vi "Audio Analysis.vi"() -> ()   [LabVIEW 2023]
doc: "演示在LabVIEW中使用队列消息处理器设计模式的基本概念。最简单的队列消息处理器由2个循环组成。“事件处理”循环通过消息队列，将用户界面事件排序为消息队列。这些消息在“消息处理”循环中出队列。注意，“消息处理”循环可以发送消息到自身。"
uses:
  Ctl/QMH Fundamentals - Message Cluster.ctl
  <vilib>/sound2/lvsound2.llb/Sampling Mode.ctl
  <vilib>/sound2/lvsound2.llb/Sound Data Format.ctl
  <vilib>/Analysis/3filter.llb/Filter Passband Type.ctl
  <vilib>/Analysis/5stat.llb/RMS (DBL).vi
  <vilib>/sound2/lvsound2.llb/Sound File Write Open.vi
  <vilib>/sound2/lvsound2.llb/Sound Input Read (DBL).vi
  <vilib>/sound2/lvsound2.llb/Sound File Write (DBL).vi
  <vilib>/Analysis/3filter.llb/Butterworth Filter (DBL).vi
  <vilib>/Analysis/NI_AALPro.lvlib
  <vilib>/Analysis/NI_AALBase.lvlib
  <vilib>/sound2/lvsound2.llb/Sound Output Write (DBL Single).vi
  <vilib>/sound2/lvsound2.llb/Sound Output Write (DBL).vi
panel:
  out "滤波后频谱图":cluster{"f0":dbl, "df":dbl, "magnitude":dbl[]}(graph) caption="波形图 2"
  out "滤波后信号":waveform(dbl)(graph)
  out "频谱图":cluster{"f0":dbl, "df":dbl, "magnitude":dbl[]}(graph) caption="波形图 2"
  out "原始信号":waveform(dbl)[](graph)
  in  "采集底噪":bool
  out "信噪比 (SNR)":dbl
  in  "滤波阶数":i32
  in  "采样数":i32
  in  "采样率":dbl
  out "音频文件保存地址":path
  out "主频 (Hz)":dbl
  out "幅值 (峰-峰值)":dbl
  in  "low cutoff freq: fl":dbl=0.12500000000000006 caption="低截止频率" format="%0.4f"
  in  "high cutoff freq: fh":dbl=0.45000000000000007 caption="高截止频率" format="%0.2f"
  in  "Filter Button":bool
  in  "quit":bool
  in  "输出设备ID":u32
  in  "输入设备ID":u32
  in  "空白按钮":bool
  # "声卡音频信号分析仪"
  # "时\n域\n图"
  # "滤\n波\n前"
  # "频\n谱\n图"
  # "时\n域\n图"
  # "滤\n波\n后"
  # "频\n谱\n图"
  # "设备设置"
  # "音频参数"
  # "滤波设置"
  # "音频文件保存"
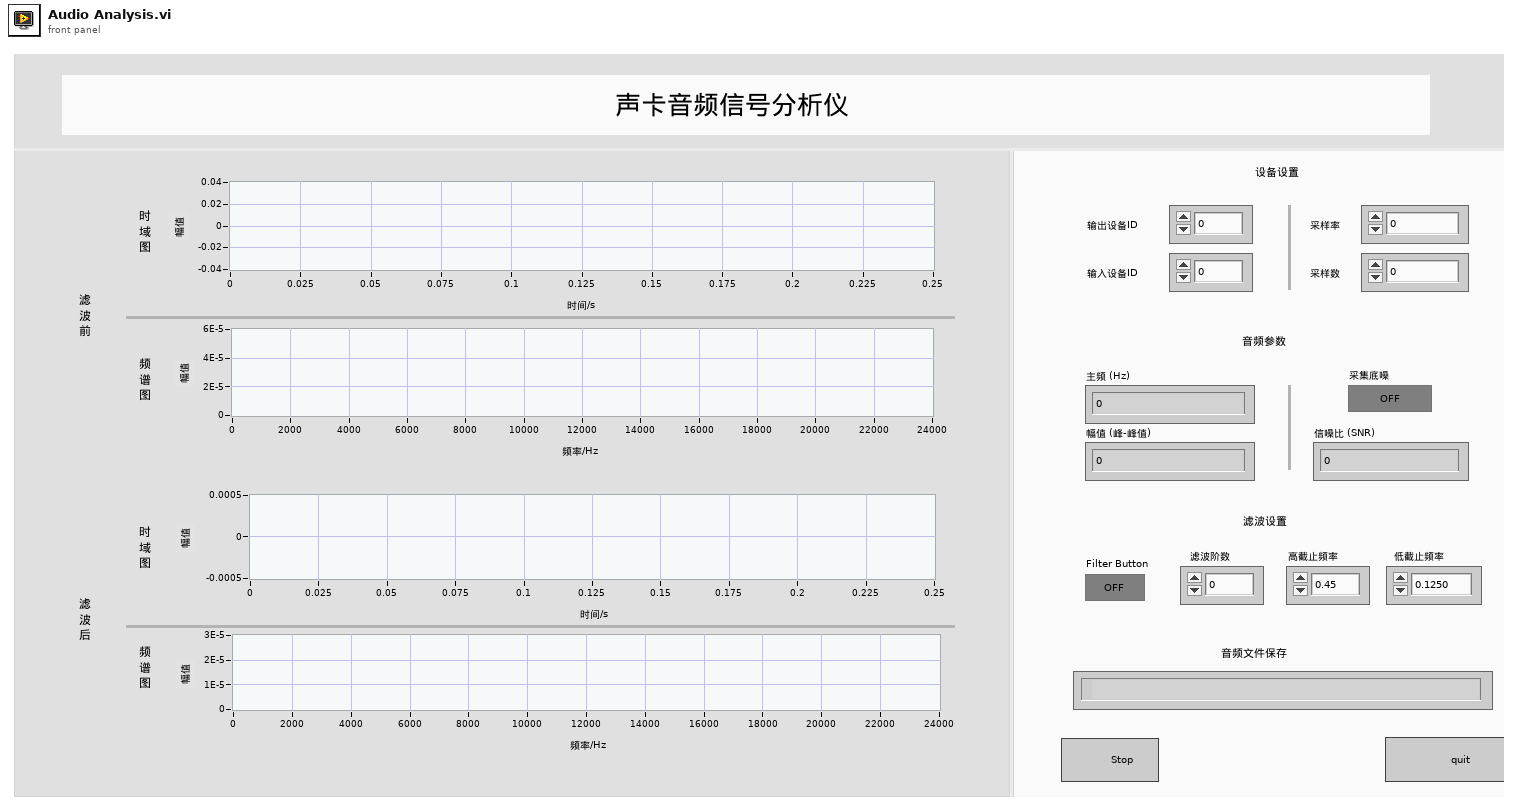
[diagram p1: front panel]
types:
  T1 = typedef "QMH Fundamentals - Message Cluster.ctl" = cluster{"消息":string, "消息数据":variant}
  T2 = typedef "Sound Data Format.ctl" = cluster{"sample rate (S/s)":dbl, "number of channels":i32, "bits per sample":i32}
  T3 = typedef "Sampling Mode.ctl" = i32
  T4 = typedef "Sound Output Task ID.ctl" = u32
  T5 = typedef "NI_AALBase.lvlib/Filter Passband Type.ctl" = enum32{"Lowpass", "Highpass", "Bandpass", "Bandstop"}
  T6 = typedef "Sound Input Task ID.ctl" = u32
  T7 = typedef "Sound File Refnum.ctl" = refnum<file>
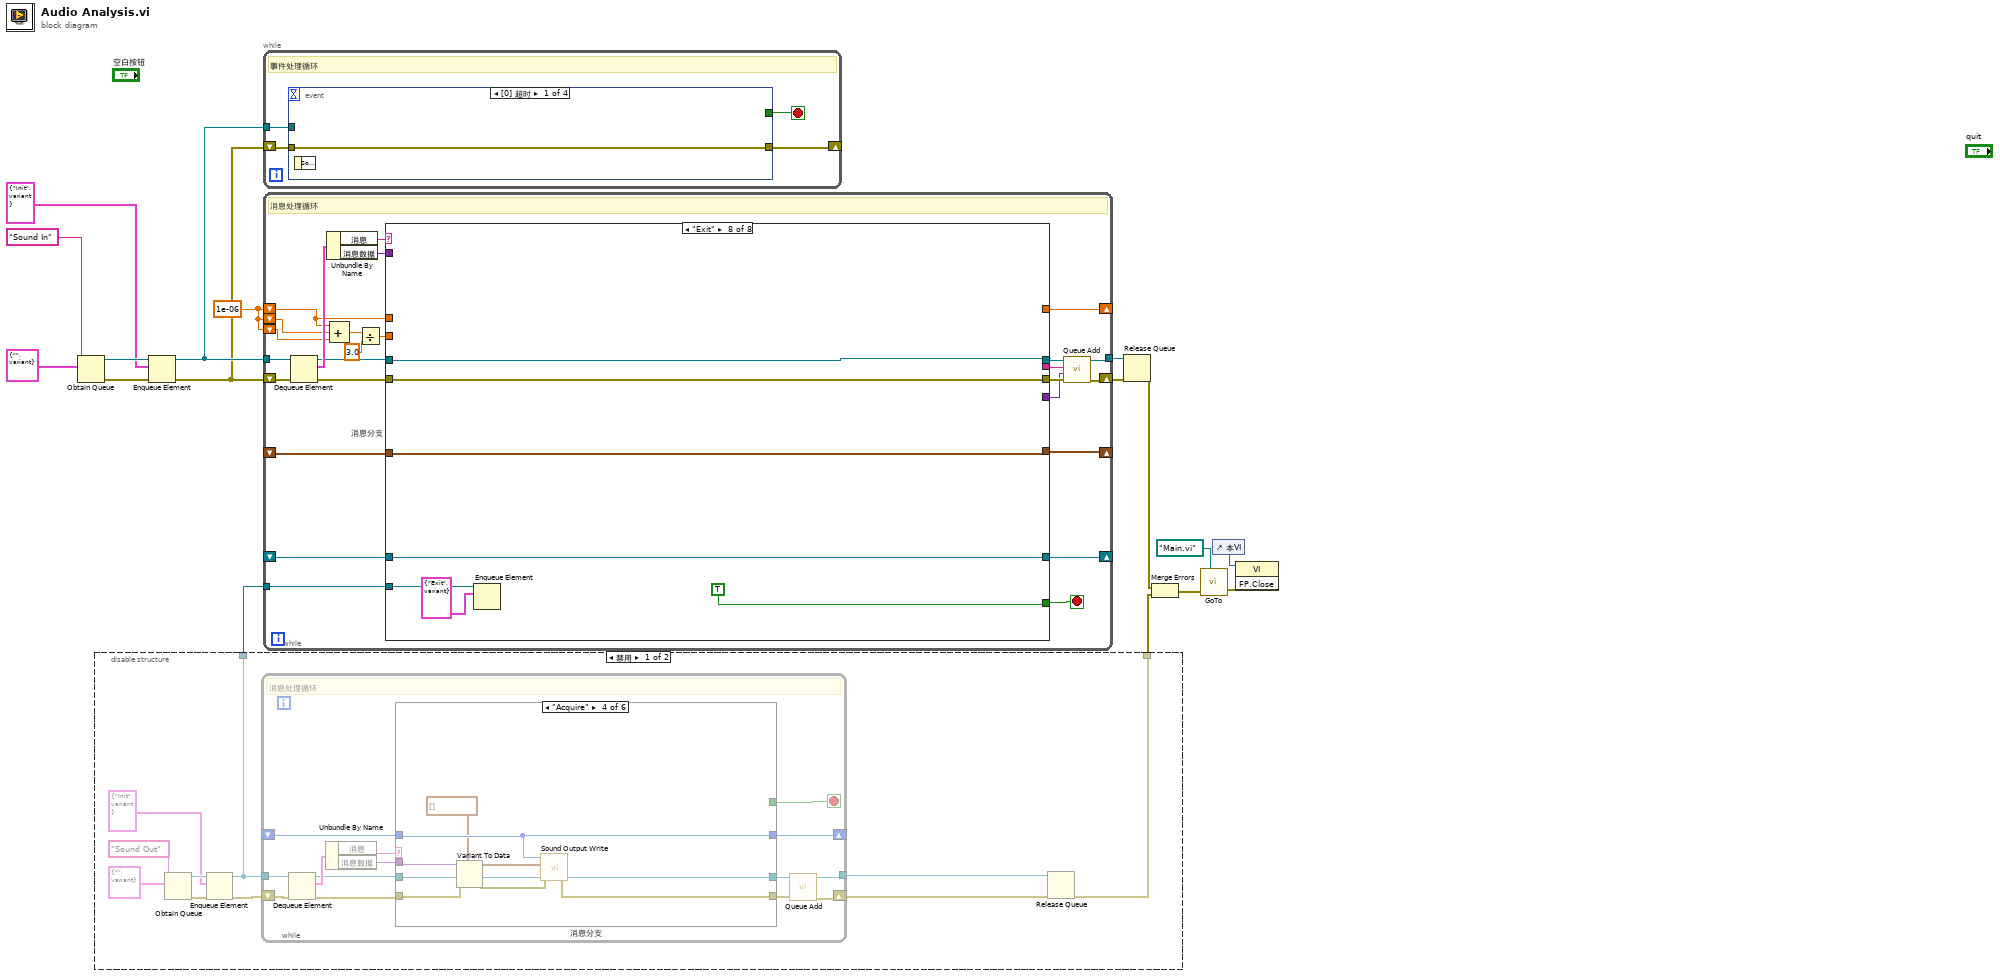
[diagram p0: block diagram]
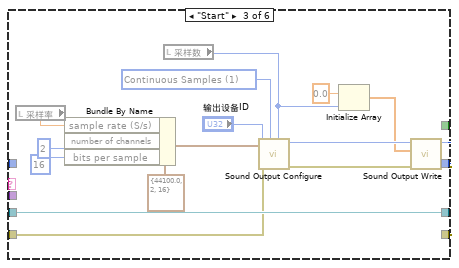
[diagram p4: hidden frame]
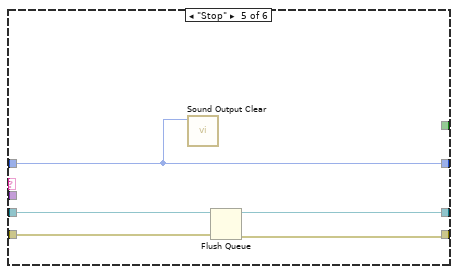
[diagram p5: hidden frame]
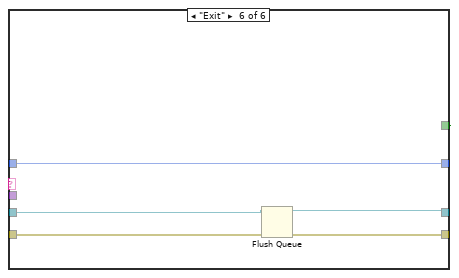
[diagram p6: hidden frame]
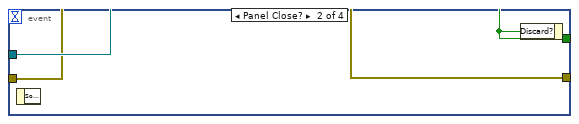
[diagram p8: hidden frame]
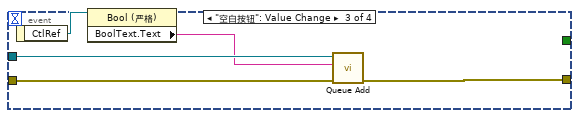
[diagram p9: hidden frame]
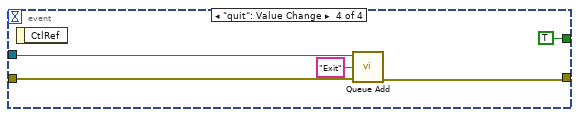
[diagram p10: hidden frame]
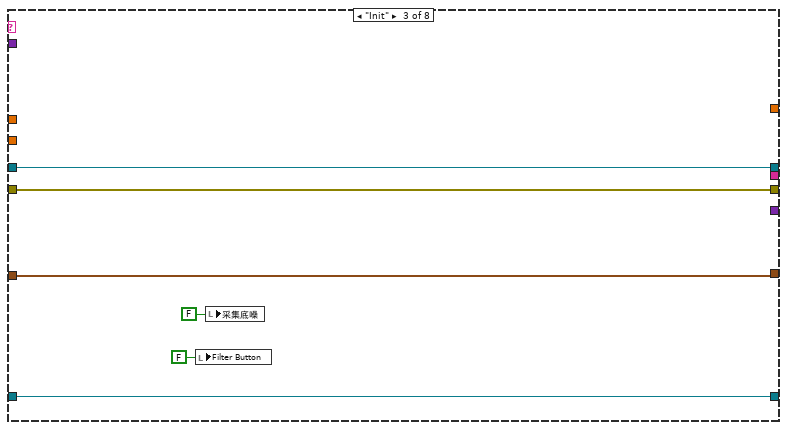
[diagram p13: hidden frame]
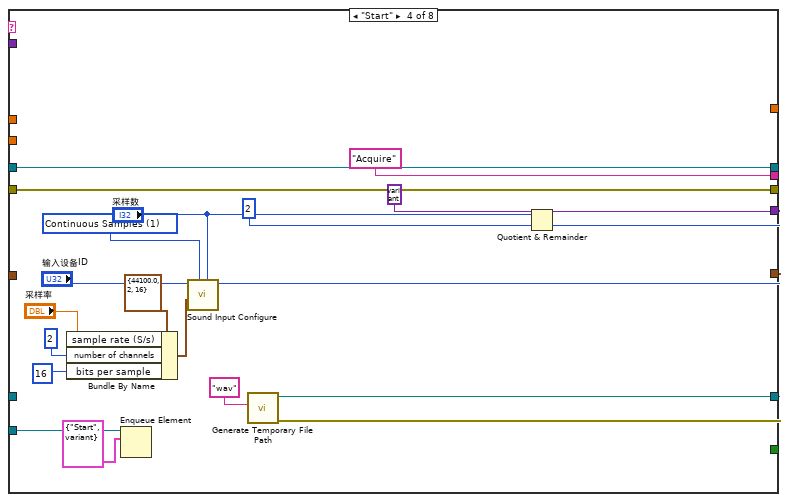
[diagram p14: hidden frame]
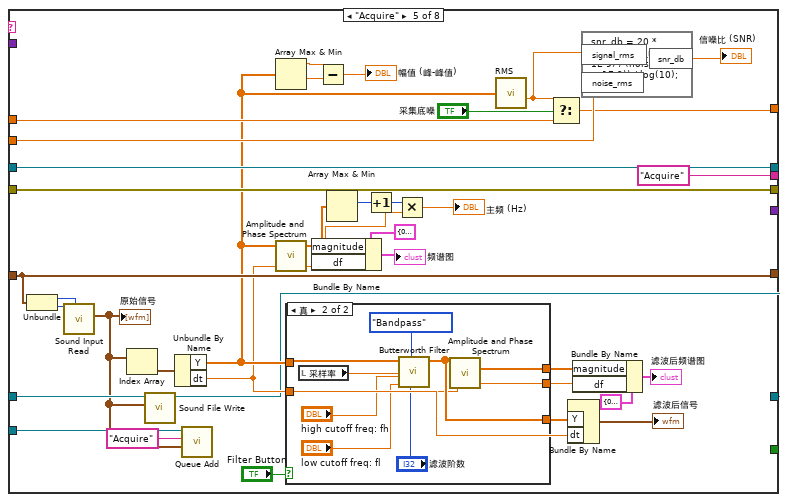
[diagram p15: hidden frame]
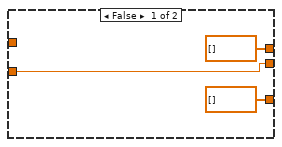
[diagram p16: hidden frame]
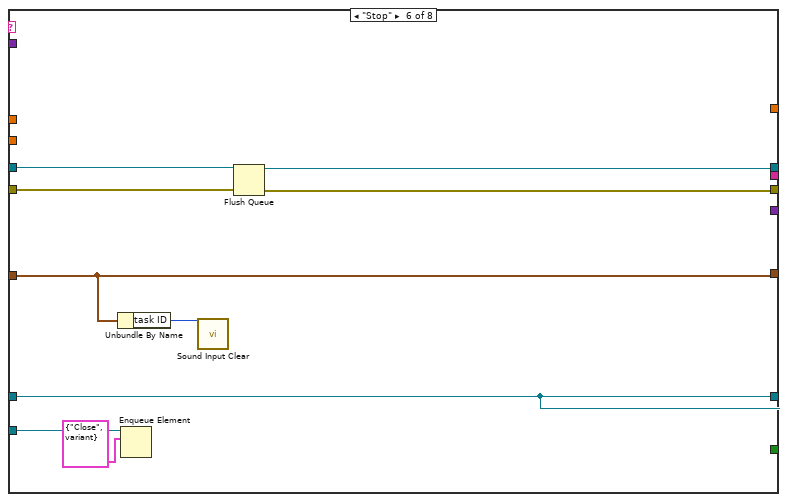
[diagram p17: hidden frame]
diagram:
  w1 = 1e-06 ("rms value")
  n1 = Obtain Queue(name (unnamed)="Sound In" ("名称（未命名）"), element data type=T1 {"消息"="", "消息数据"=variant} ("Message Cluster")) -> (queue out=w15:refnum<queue>, error out=w16:errorcluster)  [unwired: 3 in, 1 out]
  n2 = disable-structure shown="禁用" {
    disable-tunnel: [w20 _] -> w8
    disable-tunnel: [w18 _] -> w6
    frame Disabled {
      n3 = Obtain Queue(name (unnamed)="Sound Out" ("名称（未命名）"), element data type=T1 {"消息"="", "消息数据"=variant} ("Message Cluster")) -> (queue out=w21:refnum<queue>, error out=w23:errorcluster)  [unwired: 3 in, 1 out]
      n4 = Enqueue Element(queue=w21, element=T1 {"消息"="Init", "消息数据"=variant} ("元素"), error in (no error)=w23) -> (queue out=w20:refnum<queue>, error out=w26:errorcluster)  [unwired: 1 in, 1 out]
      n5 = while {
        tunnel: w20 -> [w40]
        tunnel: [w30] -> w25
        shift-right: [w29] -> w27
        shift-left: w26 -> [w41]
        shift-right: [w34] -> _
        shift-left: _ -> [w33]
        stop <- w28 stop-if-true
        # "消息处理循环"
        n6 = Dequeue Element(queue=w40, error in (no error)=w41) -> (queue out=w38:refnum<queue>, element=w39:T1, error out=w37:errorcluster)  [unwired: 1 in, 1 out]
        n7 = Unbundle By Name(w39) -> ("消息"=w36:string, "消息数据"=w35:variant)
        n8 = case "消息分支" shown="\"Acquire\"" w36 {
          tunnel: w38 -> [w43 w46 w63 w71 w75 w80]
          tunnel: w37 -> [w44 w47 w55 w66 w74 w81]
          tunnel: [w44 w47 w54 w64 w72 w78] -> w31
          tunnel: [_ _ _ _ _ TRUE] -> w28
          tunnel: w35 -> [_ _ _ w69 _ _]
          tunnel: [w43 w46 w63 w71 w73 w79] -> w32
          tunnel: [w42 w45 w56 w70 w76 w77] -> w34
          tunnel: w33 -> [w42 w45 _ w70 w76 w77]
          frame Default {
            # "初始化－执行应用的初始化代码。在本范例中所需的初始化为设置显示消息显示控件的值为空字符串。"
          }
          frame "Init" {
            # "初始化－执行应用的初始化代码。在本范例中所需的初始化为设置显示消息显示控件的值为空字符串。"
          }
          frame "Start" {
            w57 = T3 1 items=["Finite Samples", "Continuous Samples"] ("sample mode")
            n9 = local read "采样率"() -> (w49:dbl)
            n10 = Bundle By Name(cluster=T2 {"sample rate (S/s)"=44100.0, "number of channels"=2, "bits per sample"=16} ("Sound Format"), "sample rate (S/s)"=w49, "number of channels"=2, "bits per sample"=16) -> (w50:T2)
            n11 = local read "采样数"() -> (w48:i32)
            n12 = call <vilib>:"Sound Output Configure.vi"("number of samples/ch"=w48, "sample mode"=w57, "error in (no error)"=w55, "sound format"=w50, "device ID"="输出设备ID") -> ("error out"=w60:errorcluster, "task ID"=w61:T4)  [unwired: 5 in]
            n13 = Initialize Array(0.0 ("element"), w48) -> (w58:dbl[])
            n14 = call-poly <vilib>:"Sound Output Write.vi"("error in (no error)"=w60, "data"=w58, "task ID"=w61) -> ("error out"=w54:errorcluster, "task ID out"=w56:T4)  [unwired: 7 in]
          }
          frame "Acquire" {
            n15 = Variant To Data(error in=w66, type=waveform(dbl)[] [] ("data"), Variant=w69) -> (data=w67:waveform(dbl)[], error out=w65:errorcluster)
            n16 = call-poly <vilib>:"Sound Output Write.vi"("error in (no error)"=w65, "data"=w67, "task ID"=w70) -> ("error out"=w64:errorcluster)  [unwired: 7 in, 1 out]
          }
          frame "Stop" {
            n17 = call <vilib>:"Sound Output Clear.vi"("task ID"=w76) -> ()  [unwired: 10 in, 1 out]
            n18 = Flush Queue(queue=w75, error in (no error)=w74) -> (queue out=w73:refnum<queue>, error out=w72:errorcluster)  [unwired: 1 out]
          }
          frame "Exit" {
            # "退出－退出应用程序。由于此消息以优先级消息（此消息位于队列的前端）发送，且循环待停止，清理代码应在此处运行。不会处理此队列中的其他消息。"
            n19 = Flush Queue(queue=w80, error in (no error)=w81) -> (queue out=w79:refnum<queue>, error out=w78:errorcluster)  [unwired: 1 out]
          }
        }
        n20 = call "Queue Add.vi"("错误输入（无错误）"=w31, "队列输入"=w32) -> ("错误输出"=w29:errorcluster, "队列输出"=w30:refnum<queue>)  [unwired: 8 in]
      }
      n21 = Release Queue(queue=w25, error in (no error)=w27) -> (error out=w18:errorcluster)  [unwired: 1 in, 2 out]
    }
    frame Enabled {
    }
  }
  n22 = Enqueue Element(queue=w15, element=T1 {"消息"="Init", "消息数据"=variant} ("元素"), error in (no error)=w16) -> (queue out=w14:refnum<queue>, error out=w11:errorcluster)  [unwired: 1 in, 1 out]
  n23 = while {
    tunnel: w14 -> [w86]
    shift-right: [w83] -> _
    shift-left: w11 -> [w84]
    stop <- w85 stop-if-true
    # "事件处理循环"
    n24 = event shown="[0] 超时" {
      selector: _ -> [_ _ _ _]
      dyn-events: _ -> [_ _ _ _]
      timeout: _ -> [_ _ _ _]
      tunnel: [_ w92 _ TRUE ("放弃？")] -> w85
      tunnel: w86 -> [_ w91 w94 w102]
      tunnel: [w87 w89 w96 w100] -> w83
      tunnel: w84 -> [w87 w90 w95 w101]
      event Timeout {
        n25 = event-data() -> ()  [unwired: 1 in, 1 out]
      }
      event Panel Close? {
        w92 = TRUE ("放弃？")
        n26 = event-data() -> ()  [unwired: 1 in, 1 out]
        n27 = Enqueue Element(queue=w91, element=T1 {"消息"="Exit", "消息数据"=variant} ("元素"), error in (no error)=w90) -> (error out=w89:errorcluster)  [unwired: 1 in, 2 out]
        n28 = event-data("Discard?"=w92) -> ()  [unwired: 1 in, 1 out]
      }
      event "空白按钮": Value Change {
        n29 = event-data() -> ("CtlRef"=w97:refnum<vi>)  [unwired: 1 in]
        n30 = property class="Bool (严格)"(reference=w97) -> ("BoolText.Text"=w93:string)  [unwired: 1 in, 2 out]
        n31 = call "Queue Add.vi"("错误输入（无错误）"=w95, "消息"=w93, "队列输入"=w94) -> ("错误输出"=w96:errorcluster)  [unwired: 7 in, 1 out]
      }
      event "quit": Value Change {
        n32 = event-data() -> ()  [unwired: 1 in, 1 out]
        n33 = call "Queue Add.vi"("错误输入（无错误）"=w101, "消息"="Exit", "队列输入"=w102) -> ("错误输出"=w100:errorcluster)  [unwired: 7 in, 1 out]
      }
    }
  }
  n34 = while {
    tunnel: w14 -> [w126]
    tunnel: [w115] -> w12
    shift-right: [w114] -> w10
    shift-left: w11 -> [w127]
    tunnel: w8 -> [w120]
    shift-right: [w119] -> _
    shift-left: _ -> [w118]
    shift-right: [w111] -> _
    shift-left: _ -> [w110]
    shift-right: [w109] -> _
    shift-left: w1 -> [w106]
    shift-left: w1 -> [w107]
    shift-left: w1 -> [w105]
    stop <- w128 stop-if-true
    # "消息处理循环"
    n35 = Dequeue Element(queue=w126, error in (no error)=w127) -> (queue out=w124:refnum<queue>, element=w125:T1, error out=w123:errorcluster)  [unwired: 1 in, 1 out]
    n36 = Unbundle By Name(w125) -> ("消息"=w122:string, "消息数据"=w121:variant)
    n37 = Compound Arithmetic op=ADD(w106, w107, w105) -> (w104:dbl)
    n38 = Divide(x=w104, y=3.0) -> (x/y=w103:dbl)
    n39 = case "消息分支" shown="\"Exit\"" w122 {
      tunnel: w124 -> [w131 w135 w141 w163 w200 w219 w226 w234]
      tunnel: w123 -> [w132 w136 w142 w164 w201 w218 w227 w235]
      tunnel: [w132 w136 w142 w164 w201 w216 w227 w232] -> w116
      tunnel: [_ _ _ _ _ _ _ TRUE] -> w128
      tunnel: w121 -> [_ _ _ _ _ _ _ _]
      tunnel: [w131 w135 w141 w163 w200 w217 w226 w233] -> w117
      tunnel: w120 -> [_ _ _ w162 w196 w223 _ w231]
      tunnel: [w130 w134 w140 w153 w199 w221 w225 w229] -> w119
      tunnel: w118 -> [w130 w134 w140 _ w199 w221 w225 w229]
      tunnel: [_ _ _ "Acquire" ("消息") "Acquire" ("消息") _ _ _] -> w113
      tunnel: [_ _ _ variant ("消息数据") _ _ _ _] -> w112
      tunnel: [w129 w133 w139 w149 w165 w215 w224 w228] -> w111
      tunnel: w110 -> [w129 w133 w139 _ w167 w215 w224 w228]
      tunnel: [_ _ _ _ w180 _ _ _] -> w109
      tunnel: w106 -> [_ _ _ _ w182 _ _ _]
      tunnel: w103 -> [_ _ _ _ w183 _ _ _]
      frame Default {
        # "初始化－执行应用的初始化代码。在本范例中所需的初始化为设置显示消息显示控件的值为空字符串。"
      }
      frame "------------------Init------------------" {
      }
      frame "Init" {
        # "初始化－执行应用的初始化代码。在本范例中所需的初始化为设置显示消息显示控件的值为空字符串。"
        n40 = local write "Filter Button"(FALSE ("Filter Button")) -> ()
        n41 = local write "采集底噪"(FALSE ("采集底噪")) -> ()
      }
      frame "Start" {
        w155 = T3 1 items=["Finite Samples", "Continuous Samples"] ("sample mode")
        n42 = Bundle By Name(cluster=T2 {"sample rate (S/s)"=44100.0, "number of channels"=2, "bits per sample"=16} ("Sound Format"), "sample rate (S/s)"="采样率", "number of channels"=2, "bits per sample"=16) -> (w147:T2)
        n43 = Enqueue Element(queue=w162, element=T1 {"消息"="Start", "消息数据"=variant} ("元素")) -> ()  [unwired: 2 in, 3 out]
        n44 = call <vilib>:"Sound Input Configure.vi"("number of samples/ch"="采样数", "sample mode"=w155, "sound format"=w147, "device ID"="输入设备ID") -> ("task ID"=w158:T6)  [unwired: 6 in, 1 out]
        n45 = call <vilib>:"Generate Temporary File Path.vi"("Temporary File Extension (tmp)"="wav") -> ("error out"=w152:errorcluster, "Unique Temporary File Path"=w150:path)  [unwired: 9 in]
        "音频文件保存地址" <- w150
        n46 = Quotient & Remainder(x="采样数", y=2) -> (floor(x/y)=w157:i32)  [unwired: 1 out]
        n47 = Bundle(w157, "task ID"=w158) -> (w153:cluster{i32, "task ID":T6})  [unwired: 1 in]
        n48 = call-poly <vilib>:"Sound File Open.vi"("error in (no error)"=w152, "path"=w150) -> ("sound file refnum"=w149:T7)  [unwired: 8 in, 1 out]
      }
      frame "Acquire" {
        n49 = Unbundle(w199) -> (w198:i32, "task ID"=w197:T6)
        n50 = call-poly <vilib>:"Sound Input Read.vi"("number of samples/ch"=w198, "task ID"=w197) -> ("data"=w166:waveform(dbl)[])  [unwired: 7 in, 2 out]
        "原始信号" <- w166
        n51 = Index Array(array=w166) -> (element=w186:waveform(dbl))  [unwired: 1 in]
        n52 = call-poly <vilib>:"Sound File Write.vi"("data"=w166, "sound file refnum"=w167) -> ("sound file refnum out"=w165:T7)  [unwired: 8 in, 1 out]
        n53 = Unbundle By Name(w186) -> ("Y"=w174:dbl[], "dt"=w172:dbl)
        n54 = call "Queue Add.vi"("消息数据"=w166, "消息"="Acquire", "队列输入"=w196) -> ()  [unwired: 7 in, 2 out]
        n55 = Array Max & Min(array=w174) -> (max value=w187:dbl, min value=w188:dbl)  [unwired: 2 out]
        n56 = call <vilib>:"Amplitude and Phase Spectrum.vi"("dt"=w172, "Signal (V)"=w174) -> ("df"=w191:dbl, "Amp Spectrum Mag (Vrms)"=w189:dbl[])  [unwired: 1 in, 1 out]
        n57 = case shown="真" "Filter Button" {
          tunnel: [dbl[] [] ("Amp Spectrum Mag (Vrms)") w212] -> w176
          tunnel: [w202 w211] -> w175
          tunnel: w174 -> [_ w205]
          tunnel: [dbl[] [] ("Filtered X") w207] -> w173
          tunnel: w172 -> [w202 w206]
          frame False {
          }
          frame True {
            n58 = local read "采样率"() -> (w214:dbl)
            n59 = call-poly <vilib>:"Butterworth Filter.vi"("order"="滤波阶数", "filter type"=Filter_Passband_Type."Bandpass", "low cutoff freq: fl"="low cutoff freq: fl", "high cutoff freq: fh"="high cutoff freq: fh", "sampling freq: fs"=w214, "X"=w205) -> ("Filtered X"=w207:dbl[])  [unwired: 2 in, 1 out]
            n60 = call <vilib>:"Amplitude and Phase Spectrum.vi"("dt"=w206, "Signal (V)"=w207) -> ("df"=w211:dbl, "Amp Spectrum Mag (Vrms)"=w212:dbl[])  [unwired: 1 in, 1 out]
          }
        }
        n61 = Bundle By Name(cluster=cluster{"f0":dbl, "df":dbl, "magnitude":dbl[]} {"f0"=0.0, "df"=0.0, "magnitude"=[]} ("FFT - （均方根）"), "magnitude"=w189, "df"=w191) -> (→"频谱图":cluster{"f0":dbl, "df":dbl, "magnitude":dbl[]})
        n62 = Subtract(x=w187, y=w188) -> (x-y=→"幅值 (峰-峰值)":dbl)
        n63 = Array Max & Min(array=w189) -> (max index (indices)=w190:i32)  [unwired: 3 out]
        n64 = Increment(x=w190) -> (x+1=w192:i32)
        n65 = Multiply(x=w192, y=w191) -> (x*y=→"主频 (Hz)":dbl)
        n66 = call-poly <vilib>:"RMS.vi"("X"=w174) -> ("rms value"=w193:dbl)  [unwired: 1 out]
        n67 = Select(t=w193, s="采集底噪", f=w182) -> (s? t:f=w180:dbl)
        n68 = Bundle By Name("Y"=w173, "dt"=w172) -> (→"滤波后信号":waveform(dbl))  [unwired: 1 in]
        n69 = Bundle By Name(cluster=cluster{"f0":dbl, "df":dbl, "magnitude":dbl[]} {"f0"=0.0, "df"=0.0, "magnitude"=[]} ("FFT - （均方根）"), "magnitude"=w176, "df"=w175) -> (→"滤波后频谱图":cluster{"f0":dbl, "df":dbl, "magnitude":dbl[]})
        n70 = formula code="snr_db = 20 * log((signal_rms + 1E-9) / (noise_rms + 1E-9)) / log(10);"("signal_rms"=w193, "noise_rms"=w183) -> ("snr_db"=→"信噪比 (SNR)":dbl)
      }
      frame "Stop" {
        n71 = Unbundle By Name(w221) -> ("task ID"=w220:T6)
        n72 = Enqueue Element(queue=w223, element=T1 {"消息"="Close", "消息数据"=variant} ("元素")) -> ()  [unwired: 2 in, 3 out]
        n73 = call <vilib>:"Sound Input Clear.vi"("task ID"=w220) -> ()  [unwired: 10 in, 1 out]
        n74 = Flush Queue(queue=w219, error in (no error)=w218) -> (queue out=w217:refnum<queue>, error out=w216:errorcluster)  [unwired: 1 out]
        n75 = call <vilib>:"Sound File Close.vi"("sound file refnum"=w215) -> ()  [unwired: 10 in, 1 out]
      }
      frame "------------------Exit------------------" {
      }
      frame "Exit" {
        # "退出－退出应用程序。由于此消息以优先级消息（此消息位于队列的前端）发送，且循环待停止，清理代码应在此处运行。不会处理此队列中的其他消息。"
        n76 = Enqueue Element(queue=w231, element=T1 {"消息"="Exit", "消息数据"=variant} ("元素")) -> ()  [unwired: 2 in, 3 out]
        n77 = Flush Queue(queue=w234, error in (no error)=w235) -> (queue out=w233:refnum<queue>, error out=w232:errorcluster)  [unwired: 1 out]
      }
    }
    n78 = call "Queue Add.vi"("错误输入（无错误）"=w116, "消息数据"=w112, "消息"=w113, "队列输入"=w117) -> ("错误输出"=w114:errorcluster, "队列输出"=w115:refnum<queue>)  [unwired: 6 in]
  }
  n79 = Release Queue(queue=w12, error in (no error)=w10) -> (error out=w7:errorcluster)  [unwired: 1 in, 2 out]
  n80 = Merge Errors(w7, w6) -> (w4:errorcluster)
  n81 = call "GoTo.vi"("错误输入（无错误）"=w4, "名称或相对路径"=path "Main.vi") -> ("错误输出"=w2:errorcluster)  [unwired: 3 in]
  n82 = control-ref of="本VI"() -> (w5:refnum<vi>)
  n83 = invoke class="VI" method="FP.Close"(reference=w5, error in=w2) -> ()  [unwired: 1 in, 3 out]
